vi "testStreamReader.vi"(8 "error in (no error)":errorcluster, 11 "TestCase in":refnum<class "TestdotNetStreams.lvclass">) -> (0 "error out":errorcluster, 3 "TestCase out":refnum<class "TestdotNetStreams.lvclass">)   [LabVIEW 2021, in "TestdotNetStreams.lvclass"]
uses:
  TestdotNetStreams.lvclass
  <vilib>/addons/_JKI Toolkits/VI Tester/TestCase.llb/TestCase.lvclass
  C:/Program Files (x86)/National Instruments/LabVIEW 2021/vi.lib/addons/_JKI Toolkits/VI Tester/TestCase.llb/TestCase.lvclass
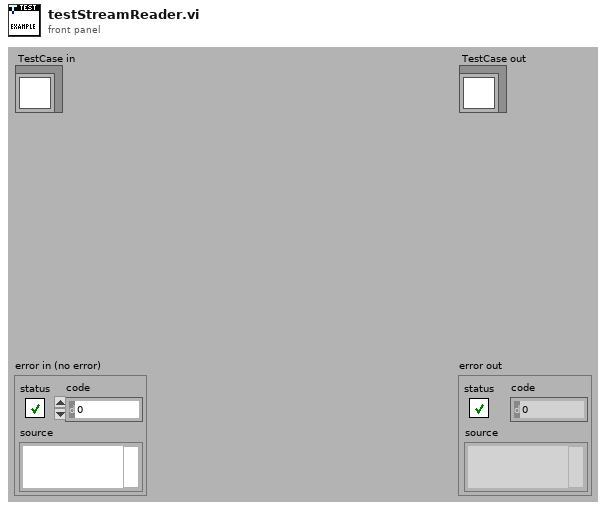
[diagram p1: front panel]
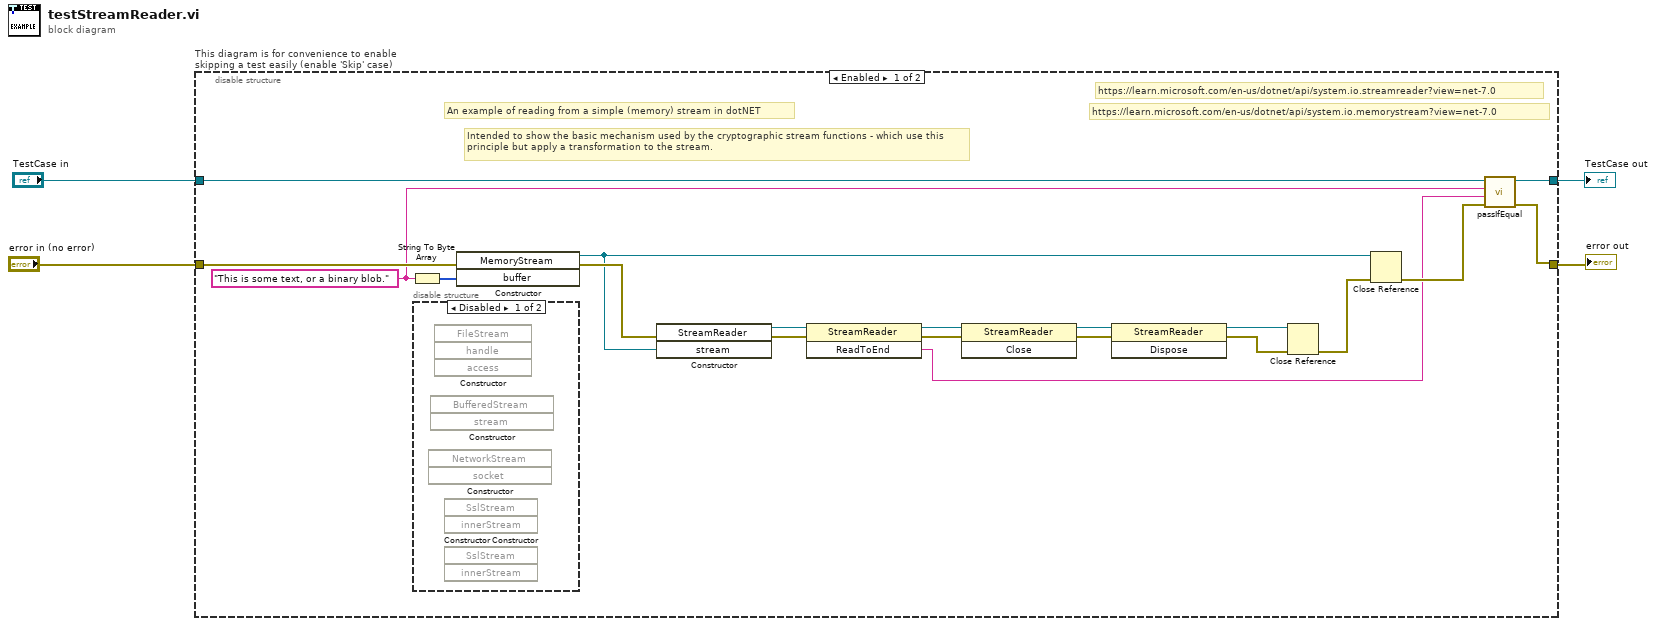
[diagram p0: block diagram]
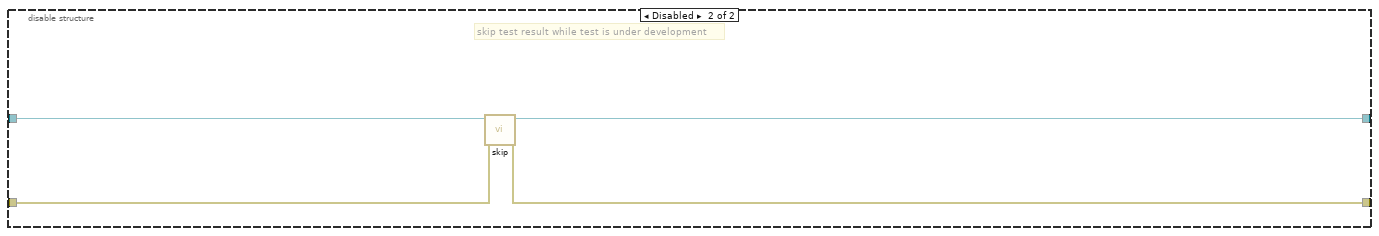
[diagram p3: hidden frame]
diagram:
  n1 = disable-structure "This diagram is for convenience to enable skipping a test easily (enable 'Skip' case)" shown="Enabled" {
    disable-tunnel: "TestCase in" -> [w23 w27]
    disable-tunnel: [w22 w25] -> w1
    disable-tunnel: [w21 w26] -> w3
    disable-tunnel: "error in (no error)" -> [w17 w24]
    frame Enabled {
      w11 = "This is some text, or a binary blob."
      # "https://learn.microsoft.com/en-us/dotnet/api/system.io.memorystream?view=net-7.0"
      # "https://learn.microsoft.com/en-us/dotnet/api/system.io.streamreader?view=net-7.0"
      # "Intended to show the basic mechanism used by the cryptographic stream functions - which use this principle but apply a transformation to the stream."
      # "An example of reading from a simple (memory) stream in dotNET"
      n2 = String To Byte Array(string=w11) -> (unsigned byte array=w12:u8[])
      n3 = disable-structure shown="Disabled" {
        frame Disabled {
          n4 = constructor class="NetworkStream"() -> ()  [unwired: 4 in, 4 out]
          n5 = constructor class="BufferedStream"() -> ()  [unwired: 4 in, 4 out]
          n6 = constructor class="FileStream"() -> ()  [unwired: 5 in, 5 out]
          n7 = constructor class="SslStream"() -> ()  [unwired: 4 in, 4 out]
          n8 = constructor class="SslStream"() -> ()  [unwired: 4 in, 4 out]
        }
        frame Enabled {
        }
      }
      n9 = constructor class="MemoryStream"(error in=w17, "buffer"=w12) -> (reference out=w15:refnum<k24>, error out=w16:errorcluster)  [unwired: 2 in, 2 out]
      n10 = constructor class="StreamReader"(error in=w16, "stream"=w15) -> (reference out=w20:refnum<k24>, error out=w19:errorcluster)  [unwired: 2 in, 2 out]
      n11 = invoke class="StreamReader" method="ReadToEnd"(reference=w20, error in=w19) -> (reference out=w9:refnum<k24>, error out=w18:errorcluster, "ReadToEnd"=w10:string)  [unwired: 1 in]
      n12 = invoke class="StreamReader" method="Close"(reference=w9, error in=w18) -> (reference out=w7:refnum<k24>, error out=w8:errorcluster)  [unwired: 1 in, 1 out]
      n13 = invoke class="StreamReader" method="Dispose"(reference=w7, error in=w8) -> (reference out=w6:refnum<k24>, error out=w5:errorcluster)  [unwired: 1 in, 1 out]
      n14 = Close Reference(reference=w6, error in (no error)=w5) -> (error out=w14:errorcluster)
      n15 = Close Reference(reference=w15, error in (no error)=w14) -> (error out=w13:errorcluster)
      n16 = call-dynamic "passIfEqual.vi"("error in (no error)"=w13, "y"=w10, "x"=w11, "TestCase in"=w23) -> ("error out"=w21:errorcluster, "TestCase out"=w22:refnum<class "TestdotNetStreams.lvclass">)  [unwired: 6 in]
    }
    frame Disabled {
      # "skip test result while test is under development"
      n17 = call <vilib>:"skip.vi"("error in (no error)"=w24, "TestCase in"=w27) -> ("error out"=w26:errorcluster, "TestCase out"=w25:refnum<class "TestdotNetStreams.lvclass">)  [unwired: 8 in]
    }
  }
  "error out" <- w3
  "TestCase out" <- w1
